vi "Direction_set.vi"(0 "VKey":T1) -> (2 "Boolean 2":bool, 3 "To/From":u16, 4 "Axis":u16)   [LabVIEW 2013]
uses:
  <vilib>/event_ctls.llb/eventvkey.ctl
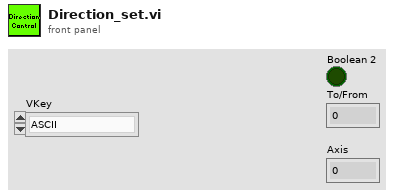
[diagram p1: front panel]
types:
  T1 = typedef "eventvkey.ctl" = enum16{"ASCII", "Enter", "Return", "Shift", "Ctrl", "Alt", "Cmd", "Opt", "Caps", "NumLock", "Clear", "Break", "Up", "Down", "Left", "Right", "Insert", "Delete", "Home", "End", "PageUp", "PageDown", "Escape", "Help", "Pause", "ScrollLock", "F1", "F2", "F3", "F4", "F5", "F6", "F7", "F8", "F9", "F10", "F11", "F12", "F13", "F14", "F15", "F16", "F17", "F18", "F19", "F20", "F21", "F22", "F23", "F24", "Play", "VolumeUp", "VolumeDown", "Mute", "Two Byte Char"}
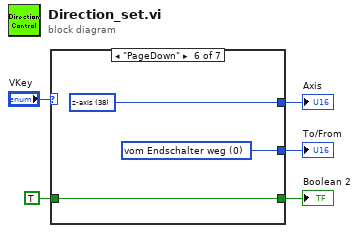
[diagram p0: block diagram]
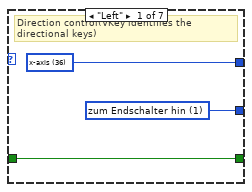
[diagram p2: hidden frame]
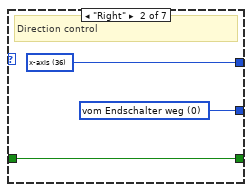
[diagram p3: hidden frame]
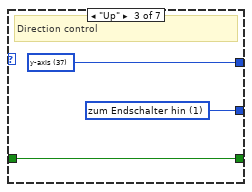
[diagram p4: hidden frame]
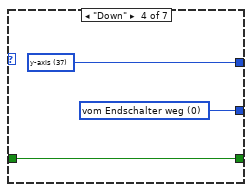
[diagram p5: hidden frame]
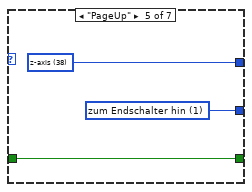
[diagram p6: hidden frame]
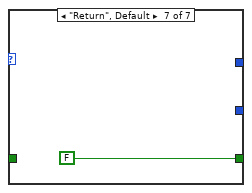
[diagram p7: hidden frame]
diagram:
  n1 = case shown="\"PageDown\"" "VKey" {
    tunnel: [w6 w9 w12 w15 w18 w21 FALSE] -> w4
    tunnel: [w8 w11 w14 w17 w20 w23 _] -> w2
    tunnel: [w7 w10 w13 w16 w19 w22 _] -> w3
    tunnel: TRUE -> [w6 w9 w12 w15 w18 w21 _]
    frame "Left" {
      w7 = u16 1 items=["vom Endschalter weg", "zum Endschalter hin"]
      w8 = u16 36 items=["x-axis"=36, "y-axis"=37, "z-axis"=38]
      # "Direction control(VKey identifies the directional keys)"
    }
    frame "Right" {
      w10 = u16 0 items=["vom Endschalter weg", "zum Endschalter hin"]
      w11 = u16 36 items=["x-axis"=36, "y-axis"=37, "z-axis"=38]
      # "Direction control"
    }
    frame "Up" {
      w13 = u16 1 items=["vom Endschalter weg", "zum Endschalter hin"]
      w14 = u16 37 items=["x-axis"=36, "y-axis"=37, "z-axis"=38]
      # "Direction control"
    }
    frame "Down" {
      w16 = u16 0 items=["vom Endschalter weg", "zum Endschalter hin"]
      w17 = u16 37 items=["x-axis"=36, "y-axis"=37, "z-axis"=38]
    }
    frame "PageUp" {
      w19 = u16 1 items=["vom Endschalter weg", "zum Endschalter hin"]
      w20 = u16 38 items=["x-axis"=36, "y-axis"=37, "z-axis"=38]
    }
    frame "PageDown" {
      w22 = u16 0 items=["vom Endschalter weg", "zum Endschalter hin"]
      w23 = u16 38 items=["x-axis"=36, "y-axis"=37, "z-axis"=38]
    }
    frame "Return", Default {
    }
  }
  "Boolean 2" <- w4
  "To/From" <- w3
  "Axis" <- w2
